vi "Inicializar Variables.vi"() -> (3 "Lista de Eventos":string[](array[string]))   [LabVIEW 2020]
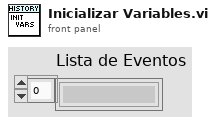
[diagram p1: front panel]
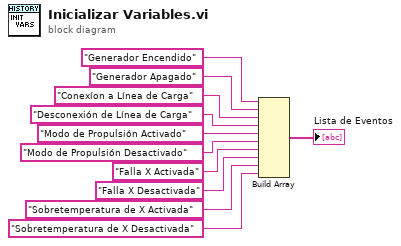
[diagram p0: block diagram]
diagram:
  n1 = Build Array("Generador Encendido", "Generador Apagado", "Conexíon a Línea de Carga", "Desconexión de Línea de Carga", "Modo de Propulsión Activado", "Modo de Propulsión Desactivado", "Falla X Activada" ("element"), "Falla X Desactivada" ("element"), "Sobretemperatura de X Activada" ("element"), "Sobretemperatura de X Desactivada" ("element")) -> (→"Lista de Eventos":string[])
